vi "Write Array of GaugeControllers.vi"(10 "Array of GaugeControllers":refnum<class "GaugeController.lvclass">[](array[class]), 11 "VacuumLines in":refnum<class "VacuumLines.lvclass">) -> (3 "VacuumLines out":refnum<class "VacuumLines.lvclass">)   [LabVIEW 2016, in "Hardware.lvlib" / "VacuumLine.lvlib" / "VacuumLines.lvclass"]
uses:
  <userlib>/Common Components/Hardware/Abstract System/VacuumLine/VacuumLines/VacuumLines.lvclass
  <userlib>/Common Components/Hardware/GaugeController/GaugeController/GaugeController.lvclass
  <userlib>/Common Components/Hardware/Abstract System/VacuumLine/VacuumLines/VacuumLines.lvclass/VacuumLines.ctl
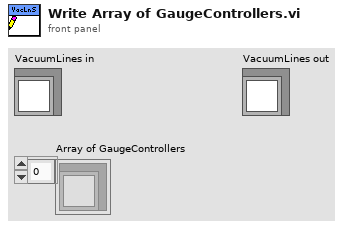
[diagram p1: front panel]
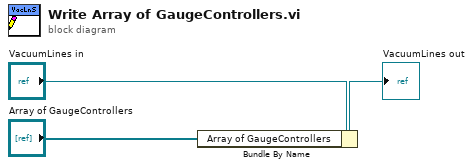
[diagram p0: block diagram]
diagram:
  n1 = Bundle By Name(cluster="VacuumLines in", "Array of GaugeControllers"="Array of GaugeControllers") -> (→"VacuumLines out":refnum<class "VacuumLines.lvclass">)
